vi "URI.vi"(11 "ErrorHandler JSON in":refnum<class "ErrorHandler JSON.lvclass">) -> (2 "URI":string, 3 "ErrorHandler JSON out":refnum<class "ErrorHandler JSON.lvclass">)   [LabVIEW 2020, in "wamplv.lvlib" / "ErrorHandler JSON.lvclass"]
uses:
  ErrorHandler JSON.lvclass
  ErrorHandler JSON.lvclass/ErrorHandler JSON.ctl
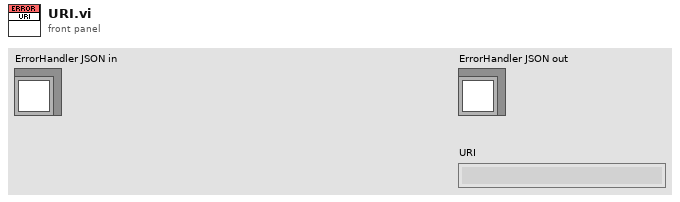
[diagram p1: front panel]
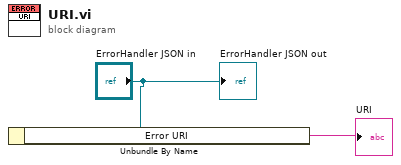
[diagram p0: block diagram]
diagram:
  n1 = Unbundle By Name("ErrorHandler JSON in") -> ("Error URI"=→"URI":string)
  "ErrorHandler JSON out" <- "ErrorHandler JSON in"
